vi "Assert Data Name Round Trip.vi"(5 "Label":string, 8 "error in (no error)":errorcluster, 10 "Variant":variant) -> (0 "error out":errorcluster, 2 "pass":bool)   [LabVIEW 2020]
uses:
  source/library/oglib_lvdata.lvlib
  <vilib>/addons/_JKI Toolkits/Caraya/classes/Assert/Assert.lvclass
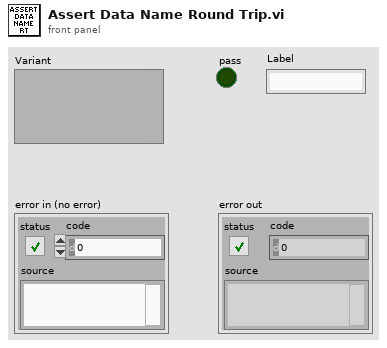
[diagram p1: front panel]
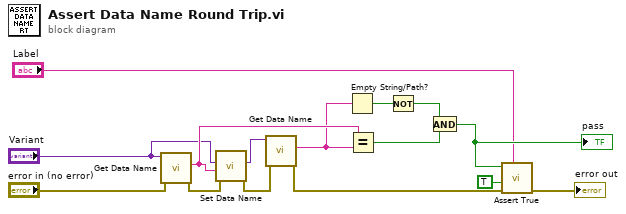
[diagram p0: block diagram]
diagram:
  n1 = call "Get Data Name.vi"("error in (no error)"="error in (no error)", "Data"="Variant") -> ("error out"=w11:errorcluster, "Data Name"=w15:string)  [unwired: 7 in, 1 out]
  n2 = call "Set Data Name.vi"("error in (no error)"=w11, "Data Name"=w15, "Data"="Variant") -> ("error out"=w13:errorcluster, "Renamed Data"=w14:variant)  [unwired: 7 in]
  n3 = call "Get Data Name.vi"("error in (no error)"=w13, "Data"=w14) -> ("error out"=w9:errorcluster, "Data Name"=w7:string)  [unwired: 7 in, 1 out]
  n4 = Empty String/Path?(string/path=w7) -> (empty?=w6:bool)
  n5 = Equal?(x=w15, y=w7) -> (x = y?=w4:bool)
  n6 = Not(x=w6) -> (.not. x?=w5:bool)
  n7 = And(x=w5, y=w4) -> (x .and. y?=w3:bool)
  "pass" <- w3
  n8 = call <vilib>:"Assert True.vi"("Label"="Label", "error in (no error)"=w9, "Register with caller test (F)"=TRUE, "True?"=w3) -> ("error out"=→"error out":errorcluster)  [unwired: 6 in, 1 out]
